vi "Calc_time.vi"(8 "Frequency":dbl, 9 "Steps on PJVS curve":i32) -> (0 "Time":i32, 1 "Frequency Out (Hz)":dbl)   [LabVIEW 2020]
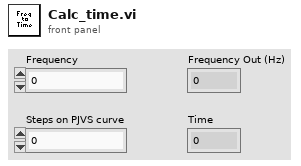
[diagram p1: front panel]
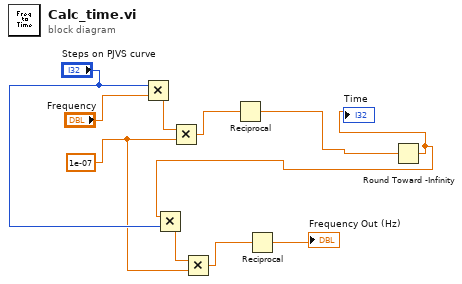
[diagram p0: block diagram]
diagram:
  w3 = 1e-07
  n1 = Multiply(x="Steps on PJVS curve", y="Frequency") -> (x*y=w9:dbl)
  n2 = Multiply(x=w9, y=w3) -> (x*y=w8:dbl)
  n3 = Reciprocal(x=w8) -> (1/x=w2:dbl)
  n4 = Round Toward -Infinity(1:w2) -> (0:w1:dbl)
  "Time" <- w1
  n5 = Multiply(x=w1, y="Steps on PJVS curve") -> (x*y=w5:dbl)
  n6 = Multiply(x=w5, y=w3) -> (x*y=w6:dbl)
  n7 = Reciprocal(x=w6) -> (1/x=→"Frequency Out (Hz)":dbl)
